vi "Init Device.vi"(8 "error in (no error)":errorcluster, 11 "NI DAQmx in":refnum<class "NI DAQmx.lvclass">) -> (0 "error out":errorcluster, 3 "NI DAQmx out":refnum<class "NI DAQmx.lvclass">)   [LabVIEW 2020, in "NI DAQmx.lvclass"]
uses:
  NI DAQmx.lvclass
  <vilib>/DAQmx/create/channels.llb/DAQmx Create Channel (DO-Digital Output).vi
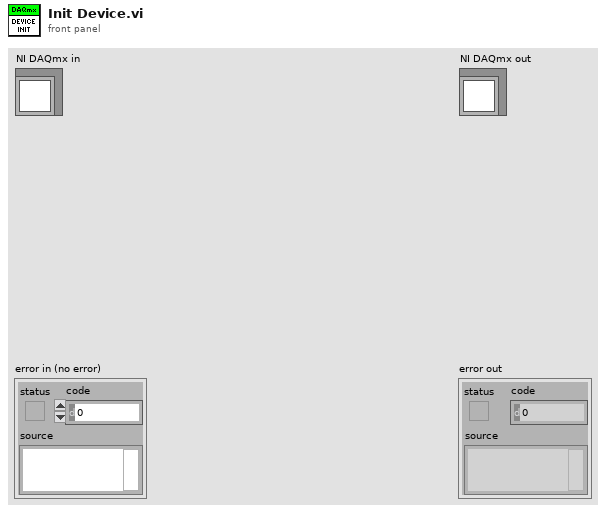
[diagram p1: front panel]
types:
  T1 = typedef "NI DAQmx.lvclass/DAQmx line name.ctl" = cluster{"lines":tag, "Function":string, "Function":enum16{"Vdd", "Control 0", "Control 1", "Control 2", "Control 3"}}
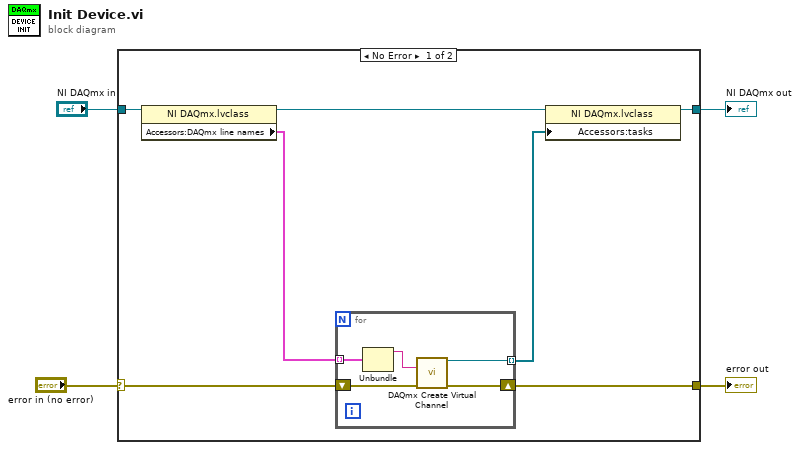
[diagram p0: block diagram]
diagram:
  n1 = case shown="No Error" "error in (no error)" {
    selector: "error in (no error)" -> [w5 w18]
    tunnel: [w9 w18] -> w3
    tunnel: [w11 w17] -> w2
    tunnel: "NI DAQmx in" -> [w6 w17]
    frame No Error {
      n2 = property class="NI DAQmx.lvclass"(reference=w6) -> (reference out=w7:refnum<class "NI DAQmx.lvclass">, "Accessors:DAQmx line names"=w8:T1[])  [unwired: 1 in, 1 out]
      n3 = for {
        tunnel: [w16] -> w10 mode=indexing
        shift-right: [w15] -> w9
        shift-left: w5 -> [w14]
        tunnel: w8 -> [w13] mode=indexing
        n4 = Unbundle(w13) -> ("lines"=w12:tag)  [unwired: 2 out]
        n5 = call-poly <vilib>:"DAQmx Create Virtual Channel.vi"("lines"=w12, "error in"=w14) -> ("task out"=w16:refnum<k21>, "error out"=w15:errorcluster)  [unwired: 12 in]
      }
      n6 = property class="NI DAQmx.lvclass"(reference=w7, "Accessors:tasks"=w10) -> (reference out=w11:refnum<class "NI DAQmx.lvclass">)  [unwired: 1 in, 1 out]
    }
    frame Error {
    }
  }
  "error out" <- w3
  "NI DAQmx out" <- w2
